vi "Build channel query command substring.vi"(0 "System no.":i32=1 min=1 max=4 step=1, 2 "Channels to query in":string[](array[string]), 3 "Query\nAll channels?":bool, 4 "For all channels: use\nChannel identifier?":bool=TRUE, 5 "error in":errorcluster, 6 "With space?":bool, 7 "Channel type":enum16{"piezo", "sensor"}(ring)) -> (14 "Command substring":string, 15 "Channels to query out":string[](array[string]), 16 "Number of rows":u32=1, 19 "error out":errorcluster)   [LabVIEW 2026]
doc: "This VI builds a query command substring for channel query commands. If Query all channels? is true, channels to command are determined in a controller specific way and returned in Channels to query out, otherwise Channels to query out is identical with Channels to query in. Number of rows is size of the Channels to query out array. If Channel identifier? is FALSE, command substring is an empty string (e.g. for systems which accept commands like VMA? without channel IDs). If With space? is true, a space character is added between the channel identifiers."
uses:
  Communication/Syntax.ctl
  GeneralCommands/Global2 (Array).vi
  Communication/Global1.vi
panel:
  # "This vi builds a query command substring for channel query commands. If \"Query all channels?\" is true, \nchannels to command are determined in a controller specific way. If \"Use axis identifier\" is false, \ncommand substring is an empty string (e.c. for VMA?). If \"With space?\" is true, a space character is added \nbetween the channel identifiers."
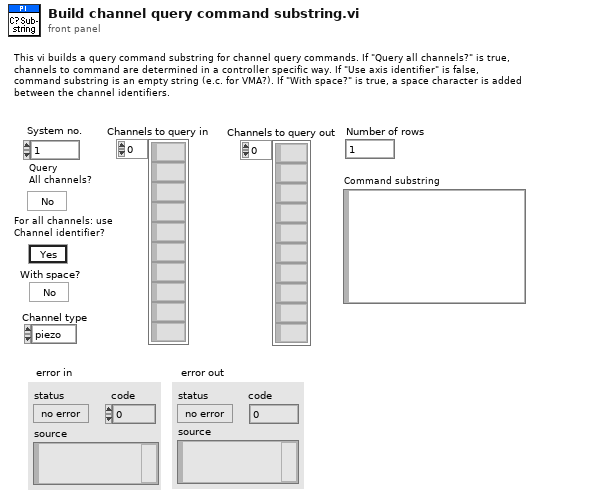
[diagram p1: front panel]
types:
  T1 = typedef "Syntax.ctl" = enum16{"GCS 1.0", "GCS 2.0", "GCS 3.0"}
  T2 = typedef "Controller names.ctl" = enum16{"None", "Analog", "C-702", "C-413", "C-414", "C-843", "C-843.PM", "C-844", "C-848", "C-865", "C-866", "C-867", "C-877", "C-880", "C-884", "C-885", "C-886", "C-887", "C-891", "E-135", "E-516", "E-517", "E-518", "E-709", "E-710", "E-712", "E-725", "E-727", "E-753", "E-754", "E-755", "E-761", "E-816", "E-861", "E-870", "E-871", "E-872", "E-873", "E-874", "F-206", "HydraPollux", "M-840", "M-850", "M-8X0", "Mercury", "Mercury_GCS", "PI_GCS2"}
  T3 = cluster{"Conn. axes":string[], "Controller name":T2}[]
  T4 = cluster{"Conn. axes":string[], "Controller name":T2}
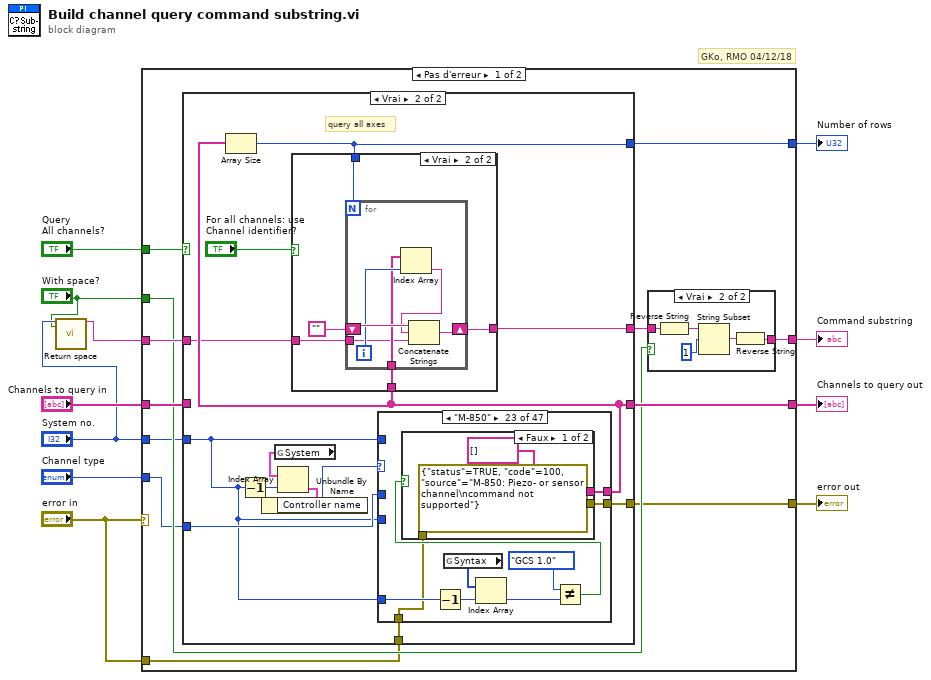
[diagram p0: block diagram]
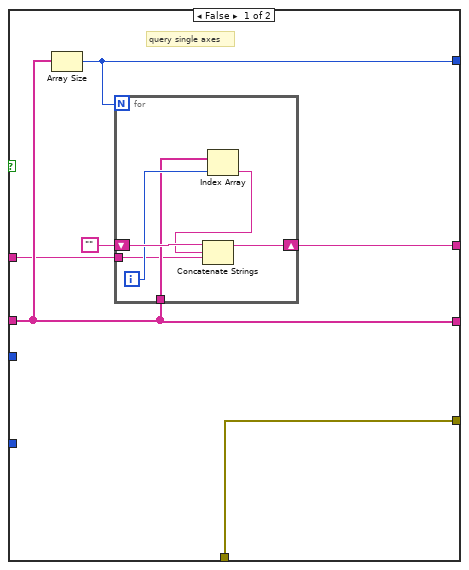
[diagram p3: hidden frame]
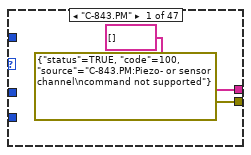
[diagram p4: hidden frame]
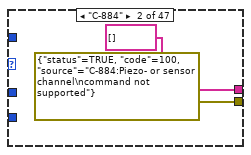
[diagram p5: hidden frame]
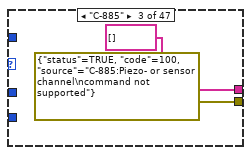
[diagram p6: hidden frame]
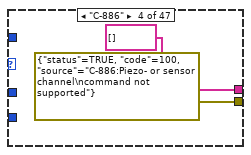
[diagram p7: hidden frame]
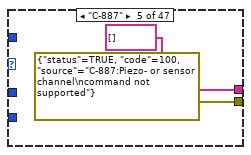
[diagram p8: hidden frame]
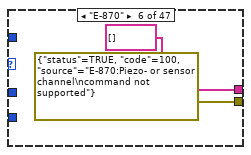
[diagram p9: hidden frame]
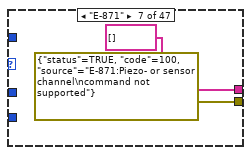
[diagram p10: hidden frame]
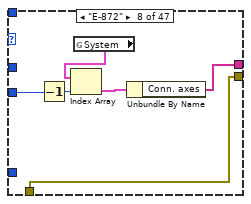
[diagram p11: hidden frame]
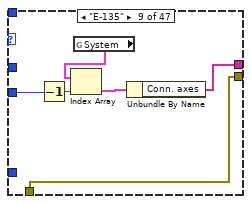
[diagram p12: hidden frame]
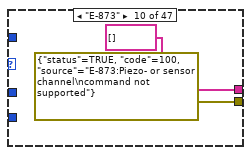
[diagram p13: hidden frame]
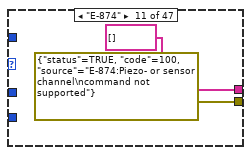
[diagram p14: hidden frame]
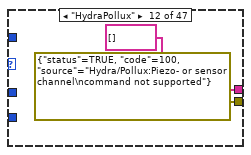
[diagram p15: hidden frame]
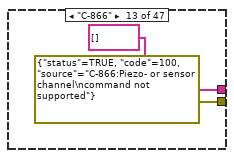
[diagram p16: hidden frame]
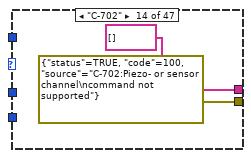
[diagram p17: hidden frame]
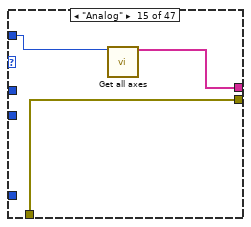
[diagram p18: hidden frame]
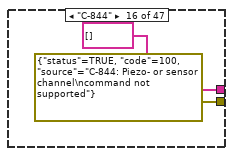
[diagram p19: hidden frame]
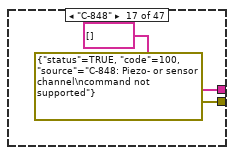
[diagram p20: hidden frame]
diagram:
  # "GKo, RMO 04/12/18"
  n1 = call "Return space.vi"("System no."="System no.", "With space?"="With space?") -> ("String out"=w3:string)  [unwired: 17 out]
  n2 = case shown="Pas d'erreur" "error in" {
    tunnel: [w23 0] -> w11
    tunnel: "Channels to query in" -> [w22 _]
    tunnel: "Query\nAll channels?" -> [w21 _]
    tunnel: [w20 string[] [] ("Axes to query in")] -> w8
    tunnel: [w19 ""] -> w7
    tunnel: w3 -> [w17 _]
    tunnel: "With space?" -> [w16 _]
    tunnel: "error in" -> [w15 w431]
    tunnel: [w14 w431] -> w6
    tunnel: "Channel type" -> [w13 _]
    tunnel: "System no." -> [w12 _]
    frame No Error {
      n3 = case shown="Vrai" w21 {
        tunnel: [w34 w54] -> w18
        tunnel: w22 -> [w33 _]
        tunnel: [w33 w51] -> w20
        tunnel: [w32 w53] -> w23
        tunnel: w17 -> [w31 w50]
        tunnel: w15 -> [w30 w49]
        tunnel: [w30 w48] -> w14
        tunnel: w13 -> [_ w47]
        tunnel: w12 -> [_ w42]
        frame False {
          # "query single axes"
          n4 = Array Size(array=w33) -> (size(s)=w32:i32)
          n5 = for {
            N: w32 -> [_]
            shift-right: [w40] -> w34
            shift-left: "" -> [w41]
            tunnel: w33 -> [w37]
            tunnel: w31 -> [w36]
            i -> [w39]
            n6 = Index Array(array=w37, index=w39) -> (element=w38:string)
            n7 = Concatenate Strings(w41, w38, w36) -> (w40:string)
          }
        }
        frame True {
          # "query all axes"
          n8 = Decrement(x=w42) -> (x-1=w45:i32)
          n9 = global read "Global2 (Array).vi" "System"() -> (w46:T3)
          n10 = Index Array(array=w46, index=w45) -> (element=w44:T4)
          n11 = Unbundle By Name(w44) -> ("Controller name"=w43:T2)
          n12 = case shown="\"M-850\"" w43 {
            tunnel: [string[] [] string[] [] string[] [] string[] [] string[] [] string[] [] string[] [] w71 w77 string[] [] string[] [] string[] [] string[] [] string[] [] w92 string[] [] string[] [] string[] [] string[] [] string[] [] w112 w125 w138 w151 string[] [] string[] [] string[] [] string[] [] string[] [] string[] [] string[] [] string[] [] w172 w179 w196 w213 w230 w247 w264 w281 w298 w315 w332 w349 w366 w383 w400] -> w51
            tunnel: w42 -> [_ _ _ _ _ _ _ w69 w75 _ _ _ _ _ _ _ _ _ _ _ _ _ _ _ _ _ _ _ _ _ _ _ w174 w183 w200 w217 w234 w251 w268 w285 w302 w319 w336 w353 w370 w387 w404]
            tunnel: w49 -> [_ _ _ _ _ _ _ w70 w76 _ _ _ _ _ w93 _ _ _ _ _ w105 w118 w131 w143 _ _ _ _ _ _ _ _ w177 w182 w199 w216 w233 w250 w267 w284 w301 w318 w335 w352 w369 w386 w403]
            tunnel: [errorcluster {"status"=TRUE, "code"=100, "source"="C-843.PM:Piezo- or sensor channel\ncommand not supported"} errorcluster {"status"=TRUE, "code"=100, "source"="C-884:Piezo- or sensor channel\ncommand not supported"} errorcluster {"status"=TRUE, "code"=100, "source"="C-885:Piezo- or sensor channel\ncommand not supported"} errorcluster {"status"=TRUE, "code"=100, "source"="C-886:Piezo- or sensor channel\ncommand not supported"} errorcluster {"status"=TRUE, "code"=100, "source"="C-887:Piezo- or sensor channel\ncommand not supported"} errorcluster {"status"=TRUE, "code"=100, "source"="E-870:Piezo- or sensor channel\ncommand not supported"} errorcluster {"status"=TRUE, "code"=100, "source"="E-871:Piezo- or sensor channel\ncommand not supported"} w70 w76 errorcluster {"status"=TRUE, "code"=100, "source"="E-873:Piezo- or sensor channel\ncommand not supported"} errorcluster {"status"=TRUE, "code"=100, "source"="E-874:Piezo- or sensor channel\ncommand not supported"} errorcluster {"status"=TRUE, "code"=100, "source"="Hydra/Pollux:Piezo- or sensor channel\ncommand not supported"} errorcluster {"status"=TRUE, "code"=100, "source"="C-866:Piezo- or sensor channel\ncommand not supported"} errorcluster {"status"=TRUE, "code"=100, "source"="C-702:Piezo- or sensor channel\ncommand not supported"} w93 errorcluster {"status"=TRUE, "code"=100, "source"="C-844: Piezo- or sensor channel\ncommand not supported"} errorcluster {"status"=TRUE, "code"=100, "source"="C-848: Piezo- or sensor channel\ncommand not supported"} errorcluster {"status"=TRUE, "code"=100, "source"="C-865: Piezo- or sensor channel\ncommand not supported"} errorcluster {"status"=TRUE, "code"=100, "source"="C-880: Piezo- or sensor channel\ncommand not supported"} errorcluster {"status"=TRUE, "code"=100, "source"="E-816: Piezo- or sensor channel\ncommand not supported"} w111 w124 w137 w150 errorcluster {"status"=TRUE, "code"=100, "source"="Mercury: Piezo- or sensor channel\ncommand not supported"} errorcluster {"status"=TRUE, "code"=100, "source"="C-843: Piezo- or sensor channel\ncommand not supported"} errorcluster {"status"=TRUE, "code"=100, "source"="None: Piezo- or sensor channel\ncommand not supported"} errorcluster {"status"=TRUE, "code"=100, "source"="Mercury_GCS: Piezo- or sensor channel\ncommand not supported"} errorcluster {"status"=TRUE, "code"=100, "source"="C-867: Piezo- or sensor channel\ncommand not supported"} errorcluster {"status"=TRUE, "code"=100, "source"="C-891: Piezo- or sensor channel\ncommand not supported"} errorcluster {"status"=TRUE, "code"=100, "source"="C-877: Piezo- or sensor channel\ncommand not supported"} errorcluster {"status"=TRUE, "code"=100, "source"="E-861: Piezo- or sensor channel\ncommand not supported"} w177 w181 w198 w215 w232 w249 w266 w283 w300 w317 w334 w351 w368 w385 w402] -> w48
            tunnel: w47 -> [_ _ _ _ _ _ _ _ _ _ _ _ _ _ _ _ _ _ _ _ _ _ _ _ _ _ _ _ _ _ _ _ _ w178 w195 w212 w229 w246 w263 w280 w297 w314 w331 w348 w365 w382 w399]
            tunnel: w42 -> [_ _ _ _ _ _ _ _ _ _ _ _ _ _ w91 _ _ _ _ _ _ _ _ _ _ _ _ _ _ _ _ _ _ _ _ _ _ _ _ _ _ _ _ _ _ _ _]
            tunnel: w42 -> [_ _ _ _ _ _ _ _ _ _ _ _ _ _ _ _ _ _ _ _ w107 w120 w133 w145 _ _ _ _ _ _ _ _ _ _ _ _ _ _ _ _ _ _ _ _ _ _ _]
            frame "C-843.PM" {
            }
            frame "C-884" {
            }
            frame "C-885" {
            }
            frame "C-886" {
            }
            frame "C-887" {
            }
            frame "E-870" {
            }
            frame "E-871" {
            }
            frame "E-872" {
              n13 = Decrement(x=w69) -> (x-1=w73:i32)
              n14 = global read "Global2 (Array).vi" "System"() -> (w74:T3)
              n15 = Index Array(array=w74, index=w73) -> (element=w72:T4)
              n16 = Unbundle By Name(w72) -> ("Conn. axes"=w71:string[])
            }
            frame "E-135" {
              n17 = Decrement(x=w75) -> (x-1=w79:i32)
              n18 = global read "Global2 (Array).vi" "System"() -> (w80:T3)
              n19 = Index Array(array=w80, index=w79) -> (element=w78:T4)
              n20 = Unbundle By Name(w78) -> ("Conn. axes"=w77:string[])
            }
            frame "E-873" {
            }
            frame "E-874" {
            }
            frame "HydraPollux" {
            }
            frame "C-866" {
            }
            frame "C-702" {
            }
            frame "Analog" {
              n21 = call "Get all axes.vi"("System no."=w91) -> ("Conn. Axes"=w92:string[])  [unwired: 18 out]
            }
            frame "C-844" {
            }
            frame "C-848" {
            }
            frame "C-865" {
            }
            frame "C-880" {
            }
            frame "E-816" {
            }
            frame "F-206" {
              n22 = Decrement(x=w107) -> (x-1=w109:i32)
              n23 = global read "Global1.vi" "Syntax"() -> (w110:T1[])
              n24 = Index Array(array=w110, index=w109) -> (element=w108:T1)
              n25 = Not Equal?(x=Syntax."GCS 1.0" ("y"), y=w108) -> (x != y?=w106:bool)
              n26 = case shown="Faux" w106 {
                tunnel: [string[] [] string[] []] -> w112
                tunnel: [errorcluster {"status"=TRUE, "code"=100, "source"="F-206: Piezo- or sensor channel\ncommand not supported"} w115] -> w111
                tunnel: w105 -> [_ w115]
                frame False {
                }
                frame True {
                }
              }
            }
            frame "M-840" {
              n27 = Decrement(x=w120) -> (x-1=w122:i32)
              n28 = global read "Global1.vi" "Syntax"() -> (w123:T1[])
              n29 = Index Array(array=w123, index=w122) -> (element=w121:T1)
              n30 = Not Equal?(x=Syntax."GCS 1.0" ("y"), y=w121) -> (x != y?=w119:bool)
              n31 = case shown="Faux" w119 {
                tunnel: [string[] [] string[] []] -> w125
                tunnel: [errorcluster {"status"=TRUE, "code"=100, "source"="M-840: Piezo- or sensor channel\ncommand not supported"} w128] -> w124
                tunnel: w118 -> [_ w128]
                frame False {
                }
                frame True {
                }
              }
            }
            frame "M-850" {
              n32 = Decrement(x=w133) -> (x-1=w135:i32)
              n33 = global read "Global1.vi" "Syntax"() -> (w136:T1[])
              n34 = Index Array(array=w136, index=w135) -> (element=w134:T1)
              n35 = Not Equal?(x=Syntax."GCS 1.0" ("y"), y=w134) -> (x != y?=w132:bool)
              n36 = case shown="Faux" w132 {
                tunnel: [string[] [] string[] []] -> w138
                tunnel: [errorcluster {"status"=TRUE, "code"=100, "source"="M-850: Piezo- or sensor channel\ncommand not supported"} w141] -> w137
                tunnel: w131 -> [_ w141]
                frame False {
                }
                frame True {
                }
              }
            }
            frame "M-8X0" {
              n37 = Decrement(x=w145) -> (x-1=w148:i32)
              n38 = global read "Global1.vi" "Syntax"() -> (w149:T1[])
              n39 = Index Array(array=w149, index=w148) -> (element=w147:T1)
              n40 = Not Equal?(x=w147, y=enum16{"GCS 1.0", "GCS 2.0"}."GCS 1.0") -> (x != y?=w144:bool)
              n41 = case shown="Faux" w144 {
                tunnel: [string[] [] string[] []] -> w151
                tunnel: [errorcluster {"status"=TRUE, "code"=100, "source"="M-8X0: Piezo- or sensor channel\ncommand not supported"} w154] -> w150
                tunnel: w143 -> [_ w154]
                frame False {
                }
                frame True {
                }
              }
            }
            frame "Mercury" {
            }
            frame "C-843" {
            }
            frame "None", Default {
            }
            frame "Mercury_GCS" {
            }
            frame "C-867" {
            }
            frame "C-891" {
            }
            frame "C-877" {
            }
            frame "E-861" {
            }
            frame "E-516" {
              n42 = Decrement(x=w174) -> (x-1=w175:i32)
              n43 = global read "Global2 (Array).vi" "System"() -> (w176:T3)
              n44 = Index Array(array=w176, index=w175) -> (element=w173:T4)
              n45 = Unbundle By Name(w173) -> ("Conn. axes"=w172:string[])
            }
            frame "E-710" {
              n46 = case shown="\"piezo\", Par défaut" w178 {
                tunnel: w183 -> [w187 w189]
                tunnel: w182 -> [w186 w190]
                tunnel: [w185 w191] -> w181
                tunnel: [w184 w188] -> w180
                frame "piezo", Default {
                  n47 = call "qTPC.vi"("System no."=w187, "error in"=w186) -> ("Number of piezo channels"=w184:i32, "error out"=w185:errorcluster)  [unwired: 16 out]
                }
                frame "sensor" {
                  n48 = call "qTSC.vi"("System no."=w189, "error in"=w190) -> ("Number of sensor channels"=w188:i32, "error out"=w191:errorcluster)  [unwired: 16 out]
                }
              }
              n49 = for {
                N: w180 -> [_]
                tunnel: [w192] -> w179 mode=indexing
                i -> [w194]
                n50 = Increment(x=w194) -> (x+1=w193:i32)
                n51 = Number To Decimal String(number=w193) -> (decimal integer string=w192:string)  [unwired: 1 out]
              }
            }
            frame "E-761" {
              n52 = case shown="\"piezo\", Par défaut" w195 {
                tunnel: w200 -> [w204 w206]
                tunnel: w199 -> [w203 w207]
                tunnel: [w202 w208] -> w198
                tunnel: [w201 w205] -> w197
                frame "piezo", Default {
                  n53 = call "qTPC.vi"("System no."=w204, "error in"=w203) -> ("Number of piezo channels"=w201:i32, "error out"=w202:errorcluster)  [unwired: 16 out]
                }
                frame "sensor" {
                  n54 = call "qTSC.vi"("System no."=w206, "error in"=w207) -> ("Number of sensor channels"=w205:i32, "error out"=w208:errorcluster)  [unwired: 16 out]
                }
              }
              n55 = for {
                N: w197 -> [_]
                tunnel: [w209] -> w196 mode=indexing
                i -> [w211]
                n56 = Increment(x=w211) -> (x+1=w210:i32)
                n57 = Number To Decimal String(number=w210) -> (decimal integer string=w209:string)  [unwired: 1 out]
              }
            }
            frame "E-755" {
              n58 = case shown="\"piezo\", Par défaut" w212 {
                tunnel: w217 -> [w221 w223]
                tunnel: w216 -> [w220 w224]
                tunnel: [w219 w225] -> w215
                tunnel: [w218 w222] -> w214
                frame "piezo", Default {
                  n59 = call "qTPC.vi"("System no."=w221, "error in"=w220) -> ("Number of piezo channels"=w218:i32, "error out"=w219:errorcluster)  [unwired: 16 out]
                }
                frame "sensor" {
                  n60 = call "qTSC.vi"("System no."=w223, "error in"=w224) -> ("Number of sensor channels"=w222:i32, "error out"=w225:errorcluster)  [unwired: 16 out]
                }
              }
              n61 = for {
                N: w214 -> [_]
                tunnel: [w226] -> w213 mode=indexing
                i -> [w228]
                n62 = Increment(x=w228) -> (x+1=w227:i32)
                n63 = Number To Decimal String(number=w227) -> (decimal integer string=w226:string)  [unwired: 1 out]
              }
            }
            frame "E-753" {
              n64 = case shown="\"piezo\", Par défaut" w229 {
                tunnel: w234 -> [w238 w240]
                tunnel: w233 -> [w237 w241]
                tunnel: [w236 w242] -> w232
                tunnel: [w235 w239] -> w231
                frame "piezo", Default {
                  n65 = call "qTPC.vi"("System no."=w238, "error in"=w237) -> ("Number of piezo channels"=w235:i32, "error out"=w236:errorcluster)  [unwired: 16 out]
                }
                frame "sensor" {
                  n66 = call "qTSC.vi"("System no."=w240, "error in"=w241) -> ("Number of sensor channels"=w239:i32, "error out"=w242:errorcluster)  [unwired: 16 out]
                }
              }
              n67 = for {
                N: w231 -> [_]
                tunnel: [w243] -> w230 mode=indexing
                i -> [w245]
                n68 = Increment(x=w245) -> (x+1=w244:i32)
                n69 = Number To Decimal String(number=w244) -> (decimal integer string=w243:string)  [unwired: 1 out]
              }
            }
            frame "E-727" {
              n70 = case shown="\"piezo\", Par défaut" w246 {
                tunnel: w251 -> [w255 w257]
                tunnel: w250 -> [w254 w258]
                tunnel: [w253 w259] -> w249
                tunnel: [w252 w256] -> w248
                frame "piezo", Default {
                  n71 = call "qTPC.vi"("System no."=w255, "error in"=w254) -> ("Number of piezo channels"=w252:i32, "error out"=w253:errorcluster)  [unwired: 16 out]
                }
                frame "sensor" {
                  n72 = call "qTSC.vi"("System no."=w257, "error in"=w258) -> ("Number of sensor channels"=w256:i32, "error out"=w259:errorcluster)  [unwired: 16 out]
                }
              }
              n73 = for {
                N: w248 -> [_]
                tunnel: [w260] -> w247 mode=indexing
                i -> [w262]
                n74 = Increment(x=w262) -> (x+1=w261:i32)
                n75 = Number To Decimal String(number=w261) -> (decimal integer string=w260:string)  [unwired: 1 out]
              }
            }
            frame "E-754" {
              n76 = case shown="\"piezo\", Par défaut" w263 {
                tunnel: w268 -> [w272 w274]
                tunnel: w267 -> [w271 w275]
                tunnel: [w270 w276] -> w266
                tunnel: [w269 w273] -> w265
                frame "piezo", Default {
                  n77 = call "qTPC.vi"("System no."=w272, "error in"=w271) -> ("Number of piezo channels"=w269:i32, "error out"=w270:errorcluster)  [unwired: 16 out]
                }
                frame "sensor" {
                  n78 = call "qTSC.vi"("System no."=w274, "error in"=w275) -> ("Number of sensor channels"=w273:i32, "error out"=w276:errorcluster)  [unwired: 16 out]
                }
              }
              n79 = for {
                N: w265 -> [_]
                tunnel: [w277] -> w264 mode=indexing
                i -> [w279]
                n80 = Increment(x=w279) -> (x+1=w278:i32)
                n81 = Number To Decimal String(number=w278) -> (decimal integer string=w277:string)  [unwired: 1 out]
              }
            }
            frame "E-709" {
              n82 = case shown="\"piezo\", Par défaut" w280 {
                tunnel: w285 -> [w289 w291]
                tunnel: w284 -> [w288 w292]
                tunnel: [w287 w293] -> w283
                tunnel: [w286 w290] -> w282
                frame "piezo", Default {
                  n83 = call "qTPC.vi"("System no."=w289, "error in"=w288) -> ("Number of piezo channels"=w286:i32, "error out"=w287:errorcluster)  [unwired: 16 out]
                }
                frame "sensor" {
                  n84 = call "qTSC.vi"("System no."=w291, "error in"=w292) -> ("Number of sensor channels"=w290:i32, "error out"=w293:errorcluster)  [unwired: 16 out]
                }
              }
              n85 = for {
                N: w282 -> [_]
                tunnel: [w294] -> w281 mode=indexing
                i -> [w296]
                n86 = Increment(x=w296) -> (x+1=w295:i32)
                n87 = Number To Decimal String(number=w295) -> (decimal integer string=w294:string)  [unwired: 1 out]
              }
            }
            frame "E-712" {
              n88 = case shown="\"sensor\"" w297 {
                tunnel: w302 -> [w306 w308]
                tunnel: w301 -> [w305 w309]
                tunnel: [w304 w310] -> w300
                tunnel: [w303 w307] -> w299
                frame "piezo", Default {
                  n89 = call "qTPC.vi"("System no."=w306, "error in"=w305) -> ("Number of piezo channels"=w303:i32, "error out"=w304:errorcluster)  [unwired: 16 out]
                }
                frame "sensor" {
                  n90 = call "qTSC.vi"("System no."=w308, "error in"=w309) -> ("Number of sensor channels"=w307:i32, "error out"=w310:errorcluster)  [unwired: 16 out]
                }
              }
              n91 = for {
                N: w299 -> [_]
                tunnel: [w311] -> w298 mode=indexing
                i -> [w313]
                n92 = Increment(x=w313) -> (x+1=w312:i32)
                n93 = Number To Decimal String(number=w312) -> (decimal integer string=w311:string)  [unwired: 1 out]
              }
            }
            frame "PI_GCS2" {
              n94 = case shown="\"sensor\"" w314 {
                tunnel: w319 -> [w323 w325]
                tunnel: w318 -> [w322 w326]
                tunnel: [w321 w327] -> w317
                tunnel: [w320 w324] -> w316
                frame "piezo", Default {
                  n95 = call "qTPC.vi"("System no."=w323, "error in"=w322) -> ("Number of piezo channels"=w320:i32, "error out"=w321:errorcluster)  [unwired: 16 out]
                }
                frame "sensor" {
                  n96 = call "qTSC.vi"("System no."=w325, "error in"=w326) -> ("Number of sensor channels"=w324:i32, "error out"=w327:errorcluster)  [unwired: 16 out]
                }
              }
              n97 = for {
                N: w316 -> [_]
                tunnel: [w328] -> w315 mode=indexing
                i -> [w330]
                n98 = Increment(x=w330) -> (x+1=w329:i32)
                n99 = Number To Decimal String(number=w329) -> (decimal integer string=w328:string)  [unwired: 1 out]
              }
            }
            frame "C-413" {
              n100 = case shown="\"piezo\", Par défaut" w331 {
                tunnel: w336 -> [w340 w342]
                tunnel: w335 -> [w339 w343]
                tunnel: [w338 w344] -> w334
                tunnel: [w337 w341] -> w333
                frame "piezo", Default {
                  n101 = call "qTPC.vi"("System no."=w340, "error in"=w339) -> ("Number of piezo channels"=w337:i32, "error out"=w338:errorcluster)  [unwired: 16 out]
                }
                frame "sensor" {
                  n102 = call "qTSC.vi"("System no."=w342, "error in"=w343) -> ("Number of sensor channels"=w341:i32, "error out"=w344:errorcluster)  [unwired: 16 out]
                }
              }
              n103 = for {
                N: w333 -> [_]
                tunnel: [w345] -> w332 mode=indexing
                i -> [w347]
                n104 = Increment(x=w347) -> (x+1=w346:i32)
                n105 = Number To Decimal String(number=w346) -> (decimal integer string=w345:string)  [unwired: 1 out]
              }
            }
            frame "C-414" {
              n106 = case shown="\"piezo\", Par défaut" w348 {
                tunnel: w353 -> [w357 w359]
                tunnel: w352 -> [w356 w360]
                tunnel: [w355 w361] -> w351
                tunnel: [w354 w358] -> w350
                frame "piezo", Default {
                  n107 = call "qTPC.vi"("System no."=w357, "error in"=w356) -> ("Number of piezo channels"=w354:i32, "error out"=w355:errorcluster)  [unwired: 16 out]
                }
                frame "sensor" {
                  n108 = call "qTSC.vi"("System no."=w359, "error in"=w360) -> ("Number of sensor channels"=w358:i32, "error out"=w361:errorcluster)  [unwired: 16 out]
                }
              }
              n109 = for {
                N: w350 -> [_]
                tunnel: [w362] -> w349 mode=indexing
                i -> [w364]
                n110 = Increment(x=w364) -> (x+1=w363:i32)
                n111 = Number To Decimal String(number=w363) -> (decimal integer string=w362:string)  [unwired: 1 out]
              }
            }
            frame "E-517" {
              n112 = case shown="\"sensor\"" w365 {
                tunnel: w370 -> [w374 w376]
                tunnel: w369 -> [w373 w377]
                tunnel: [w372 w378] -> w368
                tunnel: [w371 w375] -> w367
                frame "piezo", Default {
                  n113 = call "qTPC.vi"("System no."=w374, "error in"=w373) -> ("Number of piezo channels"=w371:i32, "error out"=w372:errorcluster)  [unwired: 16 out]
                }
                frame "sensor" {
                  n114 = call "qTSC.vi"("System no."=w376, "error in"=w377) -> ("Number of sensor channels"=w375:i32, "error out"=w378:errorcluster)  [unwired: 16 out]
                }
              }
              n115 = for {
                N: w367 -> [_]
                tunnel: [w379] -> w366 mode=indexing
                i -> [w381]
                n116 = Increment(x=w381) -> (x+1=w380:i32)
                n117 = Number To Decimal String(number=w380) -> (decimal integer string=w379:string)  [unwired: 1 out]
              }
            }
            frame "E-518" {
              n118 = case shown="\"sensor\"" w382 {
                tunnel: w387 -> [w391 w393]
                tunnel: w386 -> [w390 w394]
                tunnel: [w389 w395] -> w385
                tunnel: [w388 w392] -> w384
                frame "piezo", Default {
                  n119 = call "qTPC.vi"("System no."=w391, "error in"=w390) -> ("Number of piezo channels"=w388:i32, "error out"=w389:errorcluster)  [unwired: 16 out]
                }
                frame "sensor" {
                  n120 = call "qTSC.vi"("System no."=w393, "error in"=w394) -> ("Number of sensor channels"=w392:i32, "error out"=w395:errorcluster)  [unwired: 16 out]
                }
              }
              n121 = for {
                N: w384 -> [_]
                tunnel: [w396] -> w383 mode=indexing
                i -> [w398]
                n122 = Increment(x=w398) -> (x+1=w397:i32)
                n123 = Number To Decimal String(number=w397) -> (decimal integer string=w396:string)  [unwired: 1 out]
              }
            }
            frame "E-725" {
              n124 = case shown="\"piezo\", Par défaut" w399 {
                tunnel: w404 -> [w408 w410]
                tunnel: w403 -> [w407 w411]
                tunnel: [w406 w412] -> w402
                tunnel: [w405 w409] -> w401
                frame "piezo", Default {
                  n125 = call "qTPC.vi"("System no."=w408, "error in"=w407) -> ("Number of piezo channels"=w405:i32, "error out"=w406:errorcluster)  [unwired: 16 out]
                }
                frame "sensor" {
                  n126 = call "qTSC.vi"("System no."=w410, "error in"=w411) -> ("Number of sensor channels"=w409:i32, "error out"=w412:errorcluster)  [unwired: 16 out]
                }
              }
              n127 = for {
                N: w401 -> [_]
                tunnel: [w413] -> w400 mode=indexing
                i -> [w415]
                n128 = Increment(x=w415) -> (x+1=w414:i32)
                n129 = Number To Decimal String(number=w414) -> (decimal integer string=w413:string)  [unwired: 1 out]
              }
            }
          }
          n130 = Array Size(array=w51) -> (size(s)=w53:i32)
          n131 = case shown="Vrai" "For all channels: use\nChannel identifier?" {
            tunnel: ["" w418] -> w54
            tunnel: w51 -> [_ w421]
            tunnel: w53 -> [_ w419]
            tunnel: w50 -> [_ w417]
            frame False {
              # "Command without\naxis identifiers"
            }
            frame True {
              n132 = for {
                N: w419 -> [_]
                shift-right: [w426] -> w418
                shift-left: "" -> [w427]
                tunnel: w421 -> [w423]
                tunnel: w417 -> [w422]
                i -> [w425]
                n133 = Index Array(array=w423, index=w425) -> (element=w424:string)
                n134 = Concatenate Strings(w427, w424, w422) -> (w426:string)
              }
            }
          }
        }
      }
      n135 = case shown="Vrai" w16 {
        tunnel: [w24 w25] -> w19
        tunnel: w18 -> [w24 w27]
        frame False {
        }
        frame True {
          n136 = Reverse String(1:w27) -> (0:w29:string)
          n137 = String Subset(string=w29, offset (0)=1) -> (substring=w26:string)  [unwired: 1 out]
          n138 = Reverse String(1:w26) -> (0:w25:string)
        }
      }
    }
    frame Error {
    }
  }
  "Number of rows" <- w11
  "Channels to query out" <- w8
  "Command substring" <- w7
  "error out" <- w6
